vi "change CLFN properties.vi"() -> ()   [LabVIEW 2016]
uses:
  <vilib>/Utility/traverseref.llb/VI Scripting - Traverse.lvlib
  <vilib>/Utility/traverseref.llb/TRef TravTarget.ctl
panel:
  in  "ShowMod":bool=TRUE caption="Open modified diagrams"
  in  "ApplyMod":bool=TRUE caption="Apply modifications"
  in  "DynamicLibrary":bool=TRUE
  in  "Call convention":enum16{"C", "stdcall"}(ring)
  in  "LibPath":string="libpq.*"
  out "Mod":path[](array[path]) caption="Modified VIs"
  in  "AnyThread":bool=TRUE
  in  "folder":path=path "C:/dev/pq-labview/Connection"
  # "= specify path on diagram"
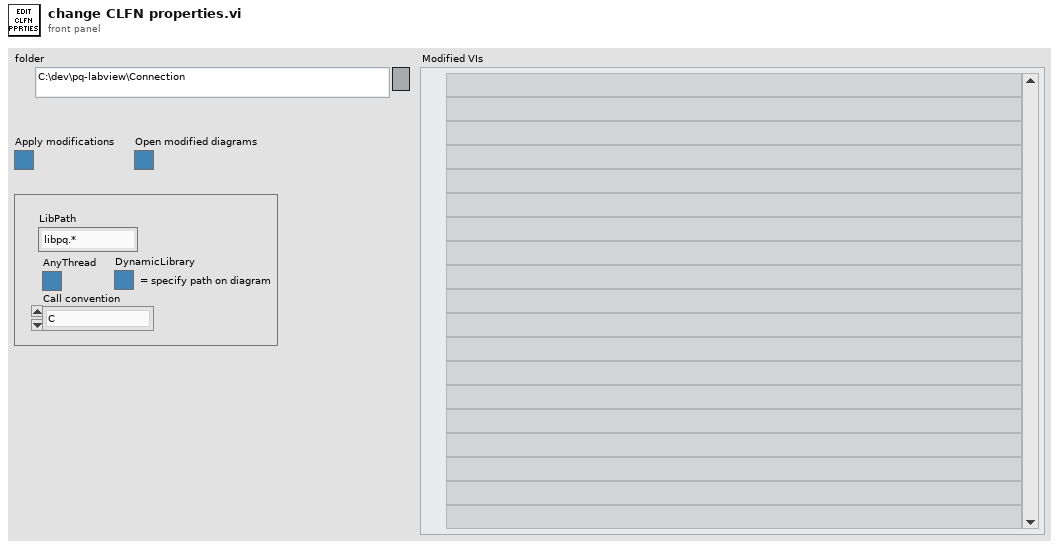
[diagram p1: front panel]
types:
  T1 = typedef "TRef TravTarget.ctl" = enum16{"FP", "BD", "Other"}
  T2 = cluster{"AnyThread":bool, path, "Calling Convention":u32, "DynamicLibrary":bool}
  T3 = cluster{"Re-entrant":bool, "LibPath":path, "CallConvention":u32, "DynamicLib":bool}
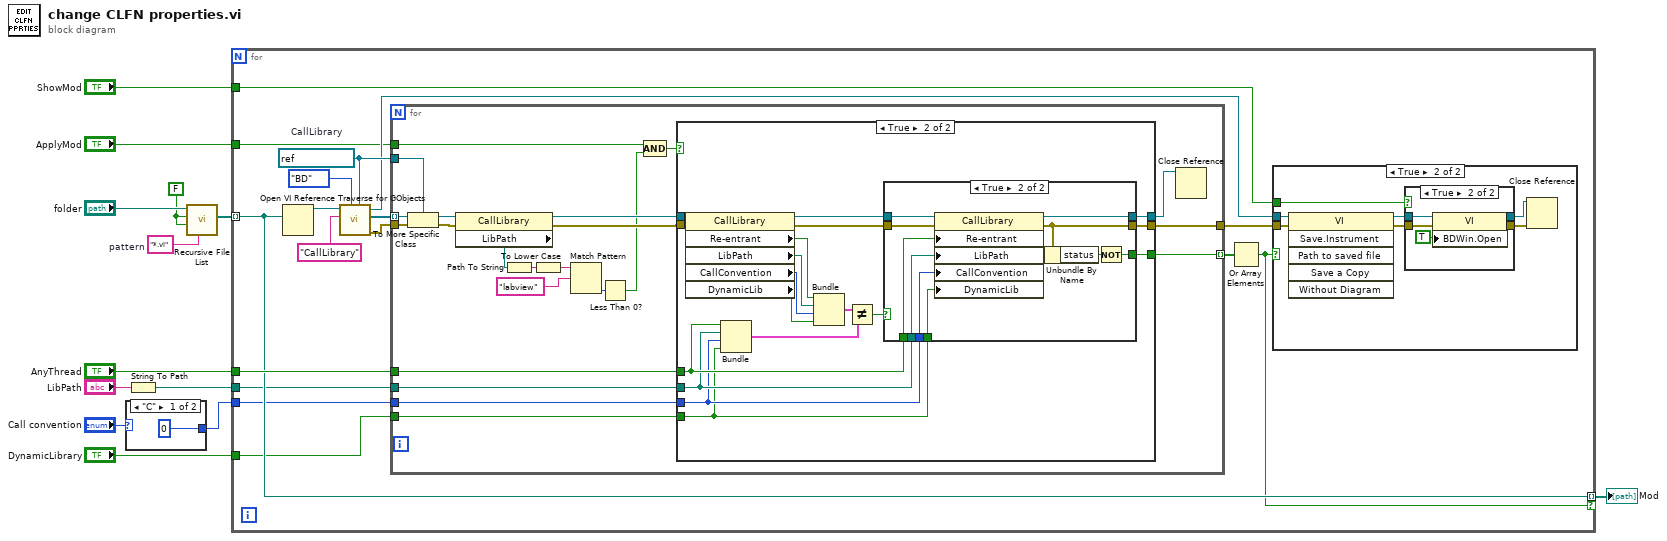
[diagram p0: block diagram]
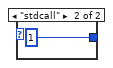
[diagram p2: hidden frame]
diagram:
  w10 = FALSE
  w9 = "*.vi"  # pattern
  n1 = case shown="\"C\"" "Call convention" {
    tunnel: [u32 0 ("Calling Convention") u32 1 ("Calling Convention")] -> w5
    frame "C" {
    }
    frame "stdcall" {
    }
  }
  n2 = String To Path(string="LibPath") -> (path=w6:path)
  n3 = call <vilib>:"Recursive File List.vi"("pattern"=w9, "Continue Recursing on Error? (F)"=w10, "Treat LLBs as Folders?"=w10, "Folder Path"="folder") -> ("All Files in Dir"=w8:path[])  [unwired: 3 in, 4 out]
  n4 = for {
    tunnel: w8 -> [w23] mode=indexing
    tunnel: "AnyThread" -> [w24]
    tunnel: [w23] -> w12 mode=indexing if=w16
    tunnel: w6 -> [w22]
    tunnel: w5 -> [w21]
    tunnel: "DynamicLibrary" -> [w20]
    tunnel: "ApplyMod" -> [w19]
    tunnel: "ShowMod" -> [w18]
    w29 = refnum<vi> refnum  # CallLibrary
    n5 = Open VI Reference(vi path=w23) -> (vi reference=w32:refnum<vi>)  [unwired: 5 in, 1 out]
    n6 = call <vilib>:"Traverse for GObjects.vi"("Other Refnum"=w29, "Traverse Target"=TRef_TravTarget."BD", "Class Name"="CallLibrary", "VI Refnum"=w32) -> ("error out"=w28:errorcluster, "References"=w25:refnum<vi>[], "dup VI Refnum"=w26:refnum<vi>)  [unwired: 4 in, 1 out]
    n7 = for {
      tunnel: w25 -> [w68] mode=indexing
      tunnel: w29 -> [w67]
      tunnel: w24 -> [w66]
      tunnel: w28 -> [w65]
      tunnel: [w64] -> w27
      tunnel: w22 -> [w63]
      tunnel: w21 -> [w61]
      tunnel: w20 -> [w60]
      tunnel: w19 -> [w59]
      tunnel: [w58] -> w17 mode=indexing
      n8 = To More Specific Class(target class=w67, reference=w68, error in=w65) -> (specific class reference=w57:refnum<vi>, error out=w56:errorcluster)
      n9 = property class="CallLibrary"(reference=w57, error in=w56) -> (reference out=w55:refnum<vi>, error out=w54:errorcluster, "LibPath"=w53:path)
      n10 = Path To String(path=w53) -> (string=w52:string)
      n11 = To Lower Case(string=w52) -> (all lower case string=w51:string)
      n12 = Match Pattern(string=w51, regular expression="labview") -> (offset past match=w49:i32)  [unwired: 1 in, 3 out]
      n13 = Less Than 0?(x=w49) -> (x < 0?=w47:bool)
      n14 = Compound Arithmetic op=AND(w59, w47) -> (w48:bool)
      n15 = case shown="True" w48 {
        tunnel: w55 -> [w70 w86]
        tunnel: w66 -> [_ w78]
        tunnel: w54 -> [w69 w83]
        tunnel: [w69 w88] -> w64
        tunnel: w63 -> [_ w77]
        tunnel: [w70 w87] -> w62
        tunnel: w61 -> [_ w76]
        tunnel: w60 -> [_ w75]
        tunnel: [_ w71] -> w58
        frame False {
        }
        frame True {
          n16 = property class="CallLibrary"(reference=w86, error in=w83) -> (reference out=w85:refnum<vi>, error out=w84:errorcluster, "Re-entrant"=w82:bool, "LibPath"=w81:path, "CallConvention"=w80:u32, "DynamicLib"=w79:bool)
          n17 = Bundle("AnyThread"=w78, w77, "Calling Convention"=w76, "DynamicLibrary"=w75) -> (w73:T2)  [unwired: 1 in]
          n18 = Bundle("Re-entrant"=w82, "LibPath"=w81, "CallConvention"=w80, "DynamicLib"=w79) -> (w74:T3)  [unwired: 1 in]
          n19 = Not Equal?(x=w74, y=w73) -> (x != y?=w72:bool)
          n20 = case shown="True" w72 {
            tunnel: [w89 w93] -> w88
            tunnel: [w90 w100] -> w87
            tunnel: w85 -> [w90 w99]
            tunnel: w84 -> [w89 w98]
            tunnel: w78 -> [_ w97]
            tunnel: w77 -> [_ w96]
            tunnel: w76 -> [_ w95]
            tunnel: w75 -> [_ w94]
            tunnel: [_ w91] -> w71
            frame False {
            }
            frame True {
              n21 = property class="CallLibrary"(reference=w99, error in=w98, "Re-entrant"=w97, "LibPath"=w96, "CallConvention"=w95, "DynamicLib"=w94) -> (reference out=w100:refnum<vi>, error out=w93:errorcluster)
              n22 = Unbundle By Name(w93) -> ("status"=w92:bool)
              n23 = Not(x=w92) -> (.not. x?=w91:bool)
            }
          }
        }
      }
      n24 = Close Reference(reference=w62) -> ()  [unwired: 1 in, 1 out]
    }
    n25 = Or Array Elements(Boolean array=w17) -> (logical OR=w16:bool)
    n26 = case shown="True" w16 {
      tunnel: w27 -> [_ w39]
      tunnel: w26 -> [_ w38]
      tunnel: w18 -> [_ w33]
      frame False {
      }
      frame True {
        n27 = invoke class="VI" method="Save.Instrument"(reference=w38, error in=w39) -> (reference out=w36:refnum<vi>, error out=w37:errorcluster)  [unwired: 4 in, 4 out]
        n28 = case shown="True" w33 {
          tunnel: w37 -> [w40 w46]
          tunnel: w36 -> [w41 w45]
          tunnel: [w41 w44] -> w35
          tunnel: [w40 w43] -> w34
          frame False {
          }
          frame True {
            n29 = property class="VI"(reference=w45, error in=w46, "BDWin.Open"=TRUE ("Block Diagram Window:Open")) -> (reference out=w44:refnum<vi>, error out=w43:errorcluster)
          }
        }
        n30 = Close Reference(reference=w35, error in (no error)=w34) -> ()  [unwired: 1 out]
      }
    }
  }
  "Mod" <- w12
